vi "HT_Contents_Measure.vi"   [LabVIEW 2014]
doc: "This \"contents\" VI contains all components of CS, which are specific for YOU, a CS user. Add your own stuff here."
uses:
  CSLebit/MM6/MM6.lvlib
  CSLebit/MM6Archiver/MM6Archiver.lvlib
  CSAcquisition/NIFPGA-MCS/NIFPGA-MCS.lvlib
  CSDigitalIO/PPG_ABC/PPG_ABC.lvlib
  CSDigitalIO/NI_FPGA_PPG/NI_FPGA_PPG.lvlib
  CSAcquisition/SR430/SR430.lvlib
  CSAcquisition/SimMCS/SimMCS.lvlib
  CSData/DiscArchiver/DiscArchiver.lvlib
  CSData/EventBuilder/EventBuilder.lvlib
  CSPentatrap/PTScanner/PTScanner.lvlib
  CSPentatrap/PTSequencer/PTSequencer.lvlib
  CSAcquisition/KE6514/KE6514.lvlib
  CSGui/KE6485GUI/KE6485GUI.lvlib
  CSGui/PPG_ABCGUI/PPG_ABCGUI.lvlib
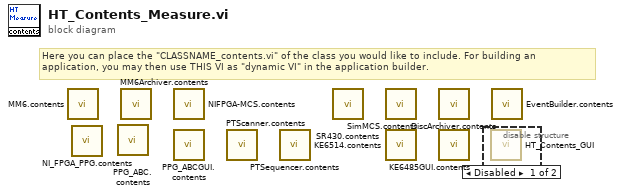
[diagram p0: block diagram]
diagram:
  # "Here you can place the \"CLASSNAME_contents.vi\" of the class you would like to include. For building an \napplication, you may then use THIS VI as \"dynamic VI\" in the application builder."
  n1 = call "MM6.contents.vi"() -> ()  [unwired: 1 in]
  n2 = call "NI_FPGA_PPG.contents.vi"() -> ()  [unwired: 1 in]
  n3 = call "PPG_ABC.contents.vi"() -> ()  [unwired: 1 in]
  n4 = call "MM6Archiver.contents.vi"() -> ()  [unwired: 1 in]
  n5 = call "NIFPGA-MCS.contents.vi"() -> ()  [unwired: 1 in]
  n6 = call "PPG_ABCGUI.contents.vi"() -> ()  [unwired: 1 in]
  n7 = call "PTScanner.contents.vi"() -> ()  [unwired: 1 in]
  n8 = call "PTSequencer.contents.vi"() -> ()  [unwired: 1 in]
  n9 = call "SR430.contents.vi"() -> ()  [unwired: 1 in]
  n10 = call "SimMCS.contents.vi"() -> ()  [unwired: 1 in]
  n11 = call "KE6514.contents.vi"() -> ()  [unwired: 20 in]
  n12 = call "DiscArchiver.contents.vi"() -> ()  [unwired: 1 in]
  n13 = call "KE6485GUI.contents.vi"() -> ()  [unwired: 20 in]
  n14 = disable-structure shown="Disabled" {
    frame Disabled {
      n15 = call "HT_Contents_GUI.vi"() -> ()  [unwired: 1 in]
    }
    frame Enabled {
    }
  }
  n16 = call "EventBuilder.contents.vi"() -> ()  [unwired: 1 in]
